vi "InitCAN.vi"(0 "DeviceType":u32, 5 "DeviceInd":u32, 7 "CANInd":u32, 9 "pInitConfig":T1, 11 "error in (no error)":errorcluster caption="错误输入（无错误）", 12 "br":u32(ring)=8 caption="波特率:" items=["Self Define", "5k bps", "10k bps", "20k bps", "40k bps", "50k bps", "80k bps", "100k bps", "125k bps", "200k bps", "250k bps", "400k bps", "500k bps", "666k bps", "800k bps", "1000k bps", "33.33k bps", "66.66k bps", "83.33k bps"]) -> (4 "Success":bool, 15 "error out":errorcluster caption="错误输出")   [LabVIEW 2011]
uses:
  data/ControlCAN.dll
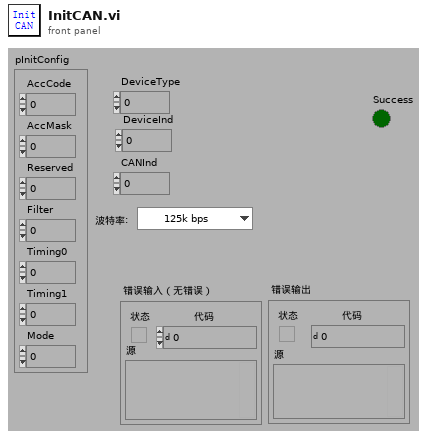
[diagram p1: front panel]
types:
  T1 = cluster{"AccCode":u32, "AccMask":u32, "Reserved":u32, "Filter":u8, "Timing0":u8, "Timing1":u8, "Mode":u8}
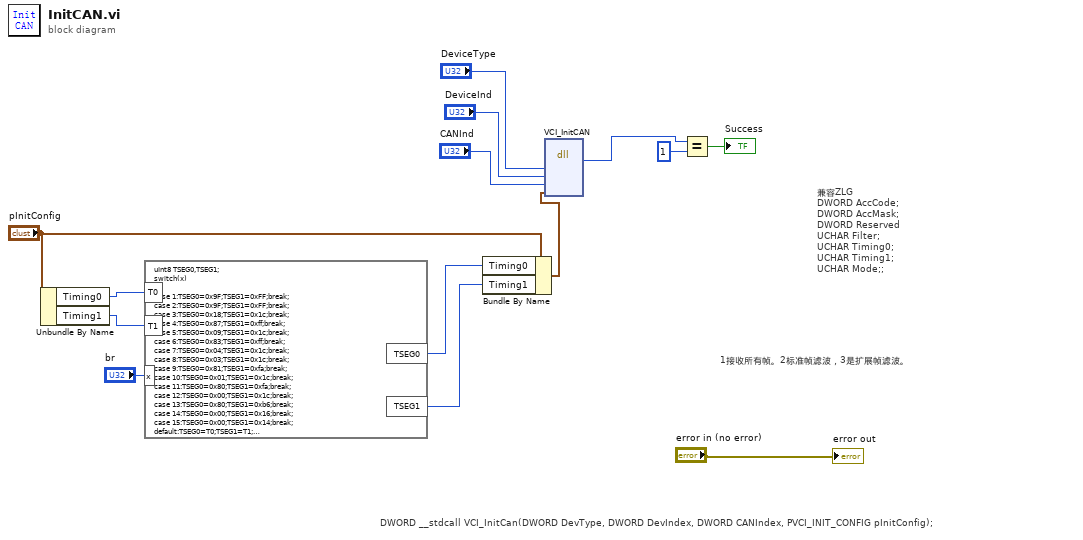
[diagram p0: block diagram]
diagram:
  # "1接收所有帧。2标准帧滤波，3是扩展帧滤波。"
  # "兼容ZLG\nDWORD AccCode;\nDWORD AccMask;\nDWORD Reserved\nUCHAR Filter;\nUCHAR Timing0;\nUCHAR Timing1;\nUCHAR Mode;;"
  # "DWORD __stdcall VCI_InitCan(DWORD DevType, DWORD DevIndex, DWORD CANIndex, PVCI_INIT_CONFIG pInitConfig);"
  n1 = Unbundle By Name("pInitConfig") -> ("Timing0"=w2:u8, "Timing1"=w1:u8)
  n2 = formula code="uInt8 TSEG0,TSEG1;\nswitch(x)\n{ \ncase 1:TSEG0=0x9F;TSEG1=0xFF;break;\ncase 2:TSEG0=0x9F;TSEG1=0xFF;break;\ncase 3:TSEG0=0x18;TSEG1=0x1c;break;\ncase 4:TSEG0=0x87;TSEG1=0xff;break;\ncase 5:TSEG0=0x09;TSEG1=0x1c;break;\ncase 6:TSEG0=0x83;TSEG1=0xff;break;\ncase 7:TSEG0=0x04;TSEG1=0x1c;break;\ncase 8:TSEG0=0x03;TSEG1=0x1c;break;\ncase 9:TSEG0=0x81;TSEG1=0xfa;break;\ncase 10:TSEG0=0x01;TSEG1=0x1c;break;\ncase 11:TSEG0=0x80;TSEG1=0xfa;break;\ncase 12:TSEG0=0x00;TSEG1=0x1c;break;\ncase 13:TSEG0=0x80;TSEG1=0xb6;break;\ncase 14:TSEG0=0x00;TSEG1=0x16;break;\ncase 15:TSEG0=0x00;TSEG1=0x14;break;\ndefault:TSEG0=T0;TSEG1=T1;\n}"("x"="br", "T0"=w2, "T1"=w1) -> ("TSEG1"=w5:u8, "TSEG0"=w6:u8)
  n3 = Bundle By Name(cluster="pInitConfig", "Timing0"=w6, "Timing1"=w5) -> (w4:T1)
  n4 = dll-call lib="PTH1Nabs D\t董海成\t上位机2.进行中USB-CAN TooldataControlCAN.dll" fn="VCI_InitCAN"("DeviceType"="DeviceType", "DeviceInd"="DeviceInd", "CANInd"="CANInd", "pInitConfig"=w4) -> ("返回类型"=w11:u32)  [unwired: 7 in, 2 out]
  n5 = Equal?(x=w11, y=u32 1) -> (x = y?=→"Success":bool)
  "error out" <- "error in (no error)"
